vi "test_Task PID Simulated Scope Simualted FGen.vi"(8 "Error In":errorcluster) -> (0 "Error Out":errorcluster)   [LabVIEW 2023]
uses:
  Task/Task Base/Task Base.lvclass
  Sample Tasks/Sample PI Control/Sample PI Control.lvclass
  Scope/Scope Simulated/Configurations/Fetch Waveforms CFG/Fetch Waveforms CFG.lvclass
  FGen/FGen Simulated/Configurations/Generate DC CFG/Generate DC CFG.lvclass
  Scope/Virtual Scopes/Virt Voltage Reader/Virt Voltage Reader.lvclass
  FGen/Virtual FGens/Virt Voltage Generator/Virt Voltage Generator.lvclass
  Task/Task Base/Task Base.lvclass/Task Base.ctl
  Measure and Stimulus Subsystems/Measure and Stimulus Subsystems.lvclass
panel:
  out "Waveform Chart Lossless":waveform(dbl)(graph)
  out "Waveform Chart Lossy":waveform(dbl)(graph)
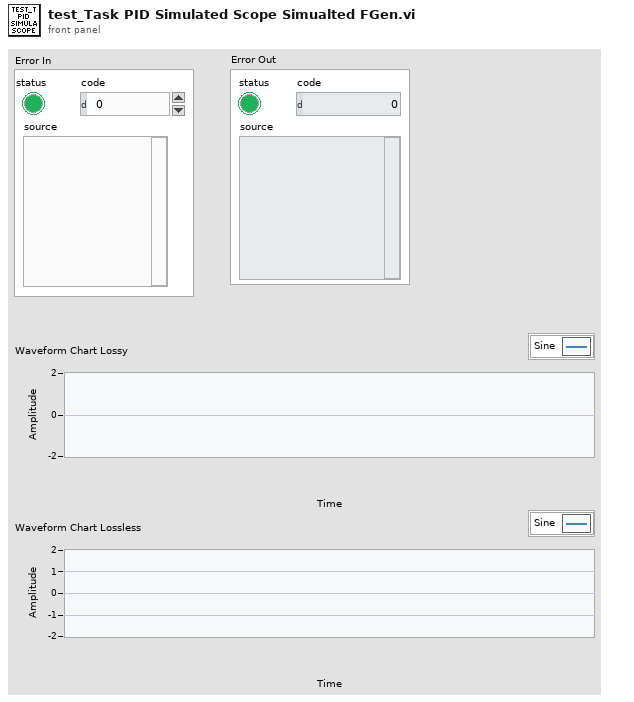
[diagram p1: front panel]
types:
  T1 = cluster{"Stop Notifier":refnum<notifier>, "Data Notifier":refnum<notifier>}
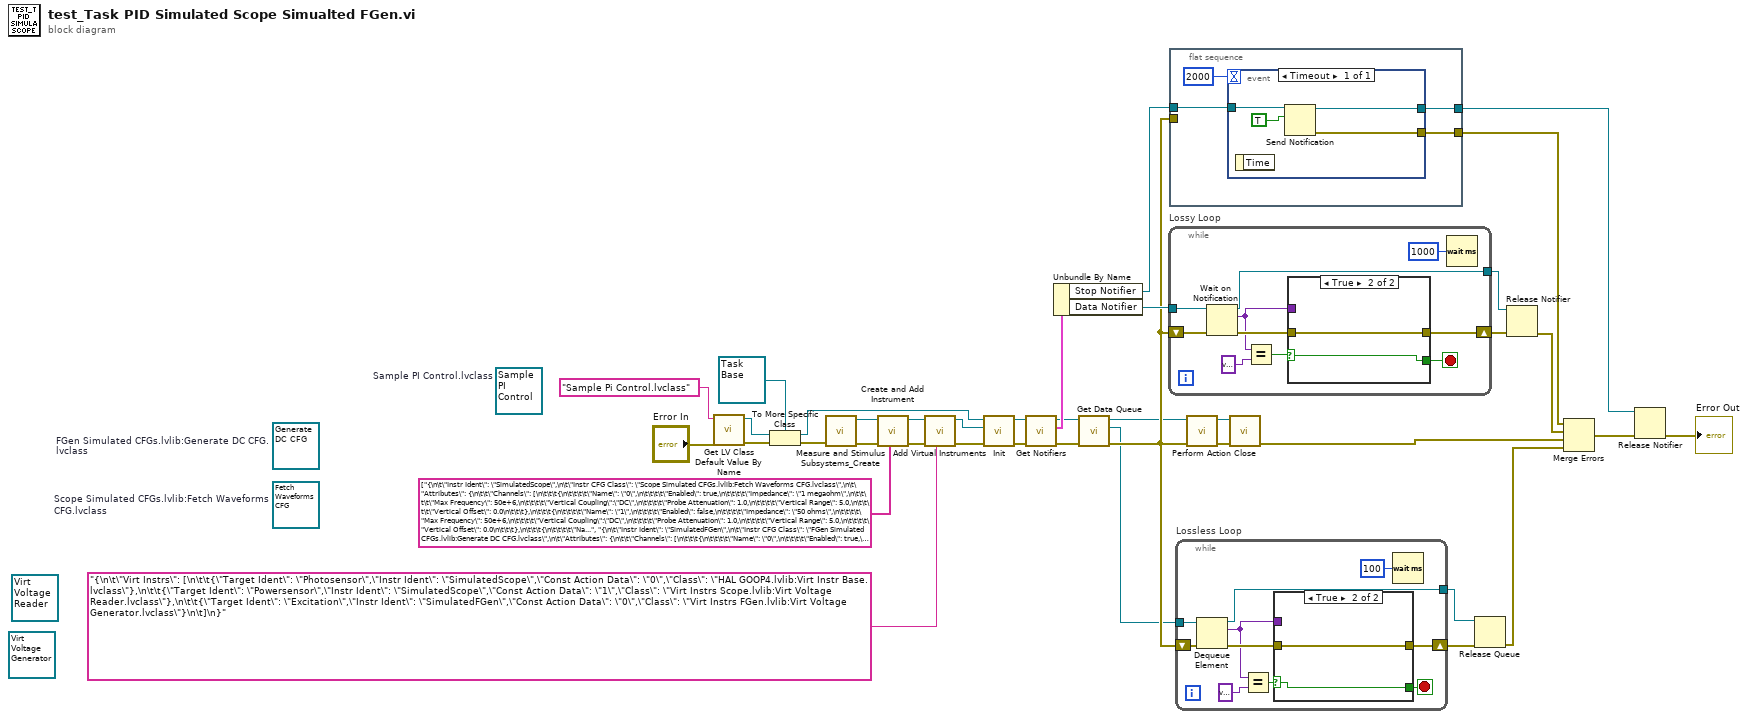
[diagram p0: block diagram]
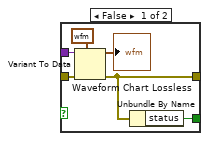
[diagram p2: hidden frame]
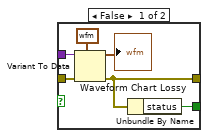
[diagram p3: hidden frame]
diagram:
  (unwired) refnum<class "Virt Voltage Generator.lvclass"> refnum ("Virt Instrs FGen.lvlib:Virt Voltage Generator.lvclass")
  (unwired) refnum<class "Virt Voltage Reader.lvclass"> refnum ("Virt Instrs Scope.lvlib:Virt Voltage Reader.lvclass")
  (unwired) refnum<class "Generate DC CFG.lvclass"> refnum  # FGen Simulated CFGs.lvlib:Generate DC CFG.lvclass
  (unwired) refnum<class "Fetch Waveforms CFG.lvclass"> refnum  # Scope Simulated CFGs.lvlib:Fetch Waveforms CFG.lvclass
  (unwired) refnum<class "Sample PI Control.lvclass"> refnum  # Sample PI Control.lvclass
  n1 = call <vilib>:"Get LV Class Default Value By Name.vi"("error in (no error)"="Error In", "class name"="Sample Pi Control.lvclass") -> ("error out"=w36:errorcluster, "object"=w33:refnum<class>)  [unwired: 8 in]
  n2 = To More Specific Class(target class=refnum<class "Task Base.lvclass"> refnum ("HAL GOOP4.lvlib:Task Base.lvclass"), reference=w33, error in=w36) -> (specific class reference=w28:refnum<class "Task Base.lvclass">, error out=w34:errorcluster)
  n3 = call "Measure and Stimulus Subsystems_Create.vi"("Error In"=w34) -> ("Error Out"=w38:errorcluster, "reference out"=w30:refnum<class "Measure and Stimulus Subsystems.lvclass">)  [unwired: 9 in]
  n4 = call "Create and Add Instrument.vi"("Physical Intr Configs"=string[] ["{\n\t\"Instr Ident\": \"SimulatedScope\",\n\t\"Instr CFG Class\": \"Scope Simulated CFGs.lvlib:Fetch Waveforms CFG.lvclass\",\n\t\"Attributes\": {\n\t\t\"Channels\": [\n\t\t\t{\n\t\t\t\t\"Name\": \"0\",\n\t\t\t\t\"Enabled\": true,\n\t\t\t\t\"Impedance\": \"1 megaohm\",\n\t\t\t\t\"Max Frequency\": 50e+6,\n\t\t\t\t\"Vertical Coupling\":\"DC\",\n\t\t\t\t\"Probe Attenuation\": 1.0,\n\t\t\t\t\"Vertical Range\": 5.0,\n\t\t\t\t\"Vertical Offset\": 0.0\n\t\t\t},\n\t\t\t{\n\t\t\t\t\"Name\": \"1\",\n\t\t\t\t\"Enabled\": false,\n\t\t\t\t\"Impedance\": \"50 ohms\",\n\t\t\t\t\"Max Frequency\": 50e+6,\n\t\t\t\t\"Vertical Coupling\":\"DC\",\n\t\t\t\t\"Probe Attenuation\": 1.0,\n\t\t\t\t\"Vertical Range\": 5.0,\n\t\t\t\t\"Vertical Offset\": 0.0\n\t\t\t},\n\t\t\t{\n\t\t\t\t\"Name\": \"2\",\n\t\t\t\t\"Enabled\": false,\n\t\t\t\t\"Impedance\": \"50 ohms\",\n\t\t\t\t\"Max Frequency\": 50e+6,\n\t\t\t\t\"Vertical Coupling\":\"DC\",\n\t\t\t\t\"Probe Attenuation\": 1.0,\n\t\t\t\t\"Vertical Range\": 5.0,\n\t\t\t\t\"Vertical Offset\": 0.0\n\t\t\t},\n\t\t\t{\n\t\t\t\t\"Name\": \"3\",\n\t\t\t\t\"Enabled\": true,\n\t\t\t\t\"Impedance\": \"50 ohms\",\n\t\t\t\t\"Max Frequency\": 50e+6,\n\t\t\t\t\"Vertical Coupling\":\"DC\",\n\t\t\t\t\"Probe Attenuation\": 1.0,\n\t\t\t\t\"Vertical Range\": 1.4,\n\t\t\t\t\"Vertical Offset\": 0.0\n\t\t\t},\n\t\t\t{\n\t\t\t\t\"Name\": \"4\",\n\t\t\t\t\"Enabled\": false,\n\t\t\t\t\"Impedance\": \"50 ohms\",\n\t\t\t\t\"Max Frequency\": 50e+6,\n\t\t\t\t\"Vertical Coupling\":\"DC\",\n\t\t\t\t\"Probe Attenuation\": 1.0,\n\t\t\t\t\"Vertical Range\": 5.0,\n\t\t\t\t\"Vertical Offset\": 0.0\n\t\t\t},\n\t\t\t{\n\t\t\t\t\"Name\": \"5\",\n\t\t\t\t\"Enabled\": false,\n\t\t\t\t\"Impedance\": \"50 ohms\",\n\t\t\t\t\"Max Frequency\": 50e+6,\n\t\t\t\t\"Vertical Coupling\":\"DC\",\n\t\t\t\t\"Probe Attenuation\": 1.0,\n\t\t\t\t\"Vertical Range\": 5.0,\n\t\t\t\t\"Vertical Offset\": 0.0\n\t\t\t},\n\t\t\t{\n\t\t\t\t\"Name\": \"6\",\n\t\t\t\t\"Enabled\": false,\n\t\t\t\t\"Impedance\": \"50 ohms\",\n\t\t\t\t\"Max Frequency\": 50e+6,\n\t\t\t\t\"Vertical Coupling\":\"DC\",\n\t\t\t\t\"Probe Attenuation\": 1.0,\n\t\t\t\t\"Vertical Range\": 5.0,\n\t\t\t\t\"Vertical Offset\": 0.0\n\t\t\t},\n\t\t\t{\n\t\t\t\t\"Name\": \"7\",\n\t\t\t\t\"Enabled\": false,\n\t\t\t\t\"Impedance\": \"50 ohms\",\n\t\t\t\t\"Max Frequency\": 50e+6,\n\t\t\t\t\"Vertical Coupling\":\"DC\",\n\t\t\t\t\"Probe Attenuation\": 1.0,\n\t\t\t\t\"Vertical Range\": 5.0,\n\t\t\t\t\"Vertical Offset\": 0.0\n\t\t\t}\n\t\t],\n\t\t\"Horizontal\": {\n\t\t\t\"Enforce Realtime\": true,\n\t\t\t\"Number of Records\": 1,\n\t\t\t\"Min Sample Rate\": 1e+5,\n\t\t\t\"Reference Position\":50, //percent\n\t\t\t\"Min Record Length\":1e+3\n\t\t},\n\t\t\"Acquire\": {\n\t\t\t\"Type\": \"Normal\",\n\t\t\t\"NumSamples\": 1e+3,\n\t\t\t\"Fetch Relative To\": \"Read Pointer\"\n\t\t},\n\t\t\"Export Signal\": {\n\t\t\t\"Signal Identifier\": \"None\",\n\t\t\t\"Signal\": \"None\",\n\t\t\t\"Output Terminal\": \"None\"\n\t\t},\n\t\t\"Trigger\": {\n\t\t\t\"Type\": \"Immediate\",\n\t\t\t\"Slope\": \"Positive\",\n\t\t\t\"Source\": \"RTSI 0\",\n\t\t\t\"Holdoff\": 0.0,\n\t\t\t\"Delay\": 0.0\n\t\t}\n\t}\n}", "{\n\t\"Instr Ident\": \"SimulatedFGen\",\n\t\"Instr CFG Class\": \"FGen Simulated CFGs.lvlib:Generate DC CFG.lvclass\",\n\t\"Attributes\": {\n\t\t\"Channels\": [\n\t\t\t{\n\t\t\t\t\"Name\": \"0\",\n\t\t\t\t\"Enabled\": true,\n\t\t\t\t\"Waveform\": \"DC\",\n\t\t\t\t\"Frequency\": 0, //DC\n\t\t\t\t\"Amplitude\": 0.0,\n\t\t\t\t\"Start Phase\": 0.0,\n\t\t\t\t\"DC Offset\": 0.0,\n\t\t\t\t\"Trigger Mode\": \"Single\"\n\t\t\t}\n\t\t],\n\t\t\"Export Signal\": {\n\t\t\t\"Enabled\": true,\n\t\t\t\"Output Terminal\": \"PFI 0\",\n\t\t\t\"Signal Identifier\": \"None\",\n\t\t\t\"Signal\": \"Start Trigger\"\n\t\t}\n\t}\n}"], "Error In"=w38, "reference in"=w30) -> ("Error Out"=w31:errorcluster, "reference out"=w29:refnum<class "Measure and Stimulus Subsystems.lvclass">)  [unwired: 7 in]
  n5 = call "Add Virtual Instruments.vi"("<JSON CFG>"="{\n\t\"Virt Instrs\": [\n\t\t{\"Target Ident\": \"Photosensor\",\"Instr Ident\": \"SimulatedScope\",\"Const Action Data\": \"0\",\"Class\": \"HAL GOOP4.lvlib:Virt Instr Base.lvclass\"},\n\t\t{\"Target Ident\": \"Powersensor\",\"Instr Ident\": \"SimulatedScope\",\"Const Action Data\": \"1\",\"Class\": \"Virt Instrs Scope.lvlib:Virt Voltage Reader.lvclass\"},\n\t\t{\"Target Ident\": \"Excitation\",\"Instr Ident\": \"SimulatedFGen\",\"Const Action Data\": \"0\",\"Class\": \"Virt Instrs FGen.lvlib:Virt Voltage Generator.lvclass\"}\n\t]\n}", "Error In"=w31, "reference in"=w29) -> ("Error Out"=w21:errorcluster, "reference out"=w27:refnum<class "Measure and Stimulus Subsystems.lvclass">)  [unwired: 7 in]
  n6 = call-dynamic "Init.vi"("error in (no error)"=w21, "MSS"=w27, "Task Base in"=w28) -> ("error out"=w10:errorcluster, "Task Base out"=w8:refnum<class "Task Base.lvclass">)  [unwired: 7 in]
  n7 = call "Get Notifiers.vi"("error in (no error)"=w10, "Task Base in"=w8) -> ("error out"=w9:errorcluster, "Notifier"=w7:T1, "Task Base out"=w3:refnum<class "Task Base.lvclass">)  [unwired: 7 in]
  n8 = Unbundle By Name(w7) -> ("Stop Notifier"=w5:refnum<notifier>, "Data Notifier"=w6:refnum<notifier>)
  n9 = call "Get Data Queue.vi"("error in (no error)"=w9, "Task Base in"=w3) -> ("error out"=w4:errorcluster, "Data Queue"=w1:refnum<queue>, "Task Base out"=w2:refnum<class "Task Base.lvclass">)  [unwired: 7 in]
  n10 = while "Lossy Loop" {
    tunnel: w6 -> [w44]
    shift-right: [w45] -> w20
    shift-left: w4 -> [w46]
    tunnel: [w43] -> w19
    stop <- w42 stop-if-true
    n11 = Wait on Notification(notifier=w44, error in (no error)=w46) -> (notifier out=w43:refnum<notifier>, notification=w40:variant, error out=w48:errorcluster)  [unwired: 2 in, 1 out]
    n12 = Equal?(x=w40, y=variant) -> (x = y?=w39:bool)
    n13 = case shown="True" w39 {
      selector: w39 -> [_ w56]
      tunnel: w48 -> [w54 w55]
      tunnel: [w52 w55] -> w45
      tunnel: [w49 w56] -> w42
      tunnel: w40 -> [w50 _]
      frame False {
        n14 = Variant To Data(error in=w54, type=waveform(dbl) {"t0"=timestamp(0 s since 1904-01-01), "dt"=1.0, "Y"=[]} ("Waveform"), Variant=w50) -> (data=→"Waveform Chart Lossy":waveform(dbl), error out=w52:errorcluster)
        n15 = Unbundle By Name(w52) -> ("status"=w49:bool)
      }
      frame True {
      }
    }
    n16 = Wait (ms)(milliseconds to wait=u32 1000) -> ()  [unwired: 1 out]
  }
  n17 = flat-sequence {
    tunnel: w4 -> [_]
    tunnel: w5 -> [w59]
    tunnel: [w58] -> w11
    tunnel: [w57] -> w14
    frame #0 {
      n18 = event shown="[0] Timeout" {
        selector: _ -> [_]
        dyn-events: _ -> [_]
        timeout: 2000 -> [_]
        tunnel: w59 -> [w64]
        tunnel: [w62] -> w58
        tunnel: [w61] -> w57
        event Timeout {
          n19 = event-data() -> ()  [unwired: 1 in, 1 out]
          n20 = Send Notification(notification=TRUE, notifier=w64) -> (notifier out=w62:refnum<notifier>, error out=w61:errorcluster)  [unwired: 1 in]
        }
      }
    }
  }
  n21 = while "Lossless Loop" {
    tunnel: w1 -> [w73]
    shift-right: [w70] -> w18
    shift-left: w4 -> [w71]
    tunnel: [w69] -> w16
    stop <- w68 stop-if-true
    n22 = Dequeue Element(queue=w73, error in (no error)=w71) -> (queue out=w69:refnum<queue>, element=w66:variant, error out=w72:errorcluster)  [unwired: 1 in, 1 out]
    n23 = Equal?(x=w66, y=variant) -> (x = y?=w65:bool)
    n24 = case shown="True" w65 {
      selector: w65 -> [_ w81]
      tunnel: w72 -> [w79 w82]
      tunnel: [w76 w82] -> w70
      tunnel: [w75 w81] -> w68
      tunnel: w66 -> [w77 _]
      frame False {
        n25 = Variant To Data(error in=w79, type=waveform(dbl) {"t0"=timestamp(0 s since 1904-01-01), "dt"=1.0, "Y"=[]} ("Waveform"), Variant=w77) -> (data=→"Waveform Chart Lossless":waveform(dbl), error out=w76:errorcluster)
        n26 = Unbundle By Name(w76) -> ("status"=w75:bool)
      }
      frame True {
      }
    }
    n27 = Wait (ms)(milliseconds to wait=u32 100) -> ()  [unwired: 1 out]
  }
  n28 = call-dynamic "Perform Action.vi"("error in (no error)"=w4, "Task Base in"=w2) -> ("error out"=w24:errorcluster, "Task Base out"=w23:refnum<class "Task Base.lvclass">)  [unwired: 7 in, 1 out]
  n29 = call-dynamic "Close.vi"("error in (no error)"=w24, "Task Base in"=w23) -> ("error out"=w22:errorcluster)  [unwired: 8 in, 1 out]
  n30 = Release Queue(queue=w16, error in (no error)=w18) -> (error out=w17:errorcluster)  [unwired: 1 in, 2 out]
  n31 = Release Notifier(notifier=w19, error in (no error)=w20) -> (error out=w13:errorcluster)  [unwired: 1 in, 2 out]
  n32 = Merge Errors(w14, w13, w22, w17) -> (w15:errorcluster)
  n33 = Release Notifier(notifier=w11, error in (no error)=w15) -> (error out=→"Error Out":errorcluster)  [unwired: 1 in, 2 out]
